vi "Calibration Helper2.vi"(7 "Std Devs":cluster{"H":dbl, "S":dbl, "V":dbl}={"H"=4.0, "S"=6.0, "V"=6.0}, 8 "Color Mode":u16(ring)=2 items=["RGB", "HSL", "HSV", "HSI", "CIE L*a*b*", "CIE XYZ"], 9 "Color Components":T1={"Hue"={110.0, 142.0}, "Sat"={138.0, 255.0}, "Val"={139.0, 198.0}} {"Val" scale=0.0..255.0; "Sat" scale=0.0..255.0; "Hue" scale=0.0..255.0 scale format="%#_3g"}, 10 "Image":T2, 11 "Image Ctl Refnum":refnum<vi>) -> (2 "Changed":bool, 3 "output color":T3)   [LabVIEW 2025]
doc: "Use the ROI (region of interest) to mask the image and compute a histogram of the indicated region. This provides the average H, S, and V values as well as the\nstandard deviation of each. It then calculates the initial upper and lower values we want to use for the threshold, and ensure that they are between 0 and 255. Hue, or the 0'th item is\na circular coordinate, so we sometimes flip the upper and lower when the computed value wraps past zero. The other values are linear and are simply clamped. This statistical approach is a reasonable approach when the ROI makes sense, but it is often useful to adjust the high/low values after the auto-calibration."
uses:
  <vilib>/vision/Image Controls.llb/IMAQ Image.ctl
  <vilib>/vision/NI_Vision_Development_Module.lvlib
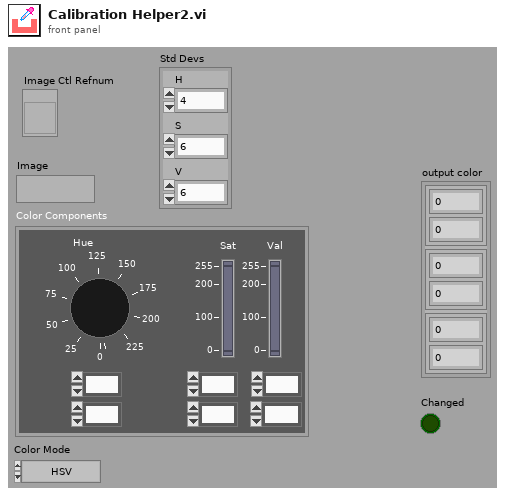
[diagram p1: front panel]
types:
  T1 = cluster{"Hue":cluster{dbl, dbl}, "Sat":cluster{dbl, dbl}, "Val":cluster{dbl, dbl}}
  T2 = typedef "IMAQ Image.ctl" = refnum<image>
  T3 = cluster{cluster{dbl, dbl}, cluster{dbl, dbl}, cluster{dbl, dbl}}
  T4 = typedef "Image Type" = u32
  T5 = cluster{"Global Rectangle":i32[], "Contours":cluster{"Contour Type":u32, "ROI Type":u32, "Points":i32[]}[]}
  T6 = cluster{"histogram":u32[], "Minimal Value":sgl, "Maximal Value":sgl, "Starting Value":sgl, "Interval Width":sgl, "Mean Value":sgl, "Standard  Variation":sgl, "Area (pixels)":i32}
  T7 = cluster{"histogram":u32[], "Minimal Value":sgl, "Maximal Value":sgl, "Starting Value":sgl, "Interval Width":sgl, "Mean Value":sgl, "Standard  Variation":sgl, "Area (pixels)":i32}[]
  T8 = cluster{"[0]":cluster{dbl, dbl}, "[1]":cluster{dbl, dbl}, "[2]":cluster{dbl, dbl}}
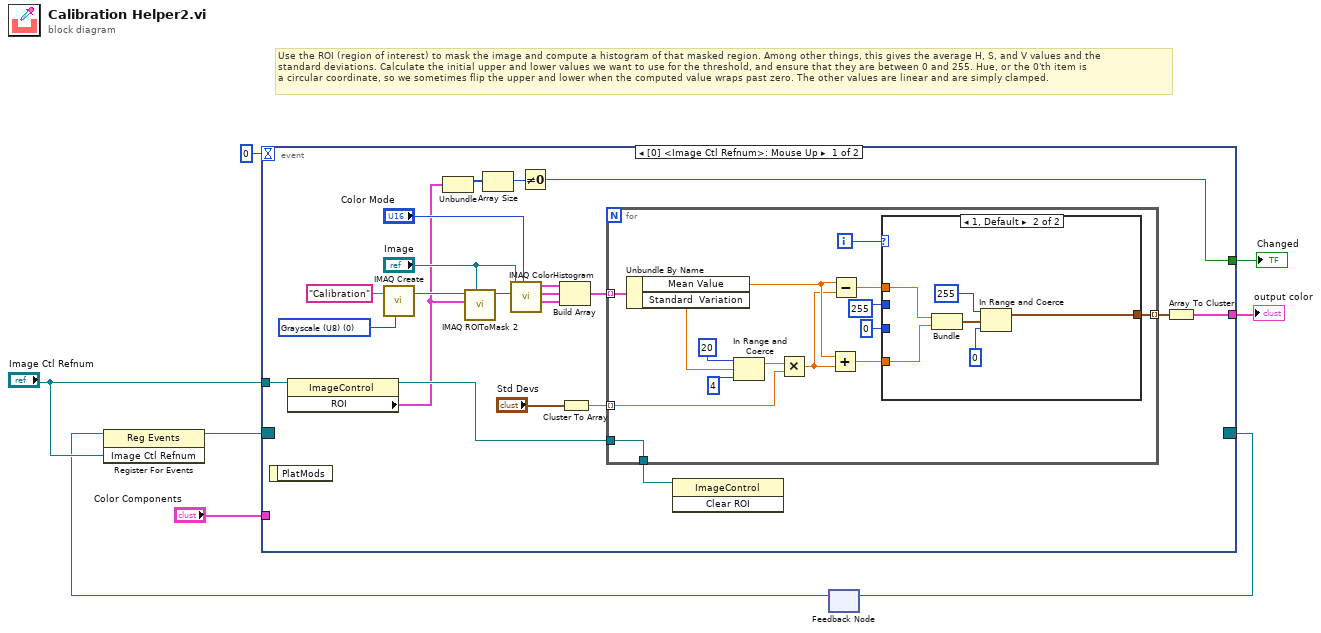
[diagram p0: block diagram]
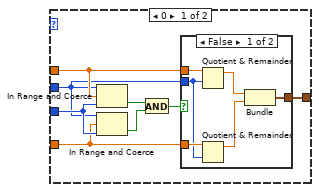
[diagram p2: hidden frame]
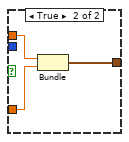
[diagram p3: hidden frame]
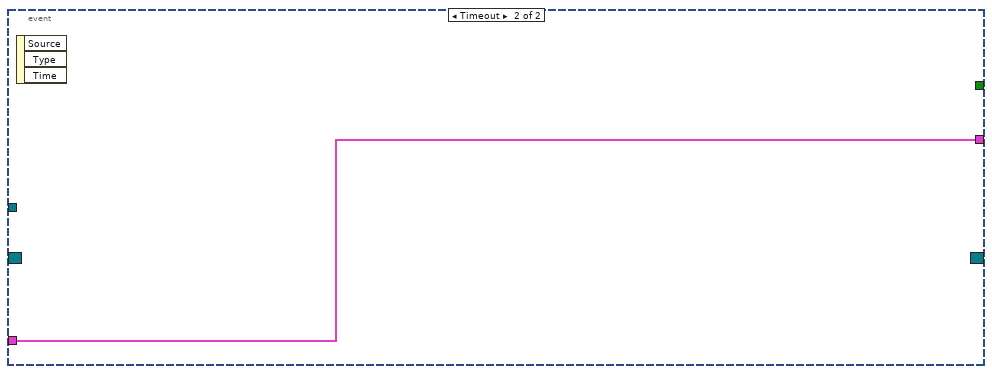
[diagram p4: hidden frame]
diagram:
  # "Use the ROI (region of interest) to mask the image and compute a histogram of that masked region. Among other things, this gives the average H, S, and V values and the\nstandard deviations. Calculate the initial upper and lower values we want to use for the threshold, and ensure that they are between 0 and 255. Hue, or the 0'th item is\na circular coordinate, so we sometimes flip the upper and lower when the computed value wraps past zero. The other values are linear and are simply clamped."
  n1 = feedback #1() -> (w2:refnum<event-registration>)  [unwired: 1 in]
  n2 = register-events(reference=w2, "Image Ctl Refnum") -> (reference out=w6:refnum<event-registration>)  [unwired: 1 in, 1 out]
  n3 = event shown="[0] <Image Ctl Refnum>: Mouse Up" {
    selector: w6 -> [_ _]
    dyn-events: [_ _] -> w3
    timeout: 0 -> [_ _]
    tunnel: "Image Ctl Refnum" -> [w16 _]
    tunnel: "Color Components" -> [_ w68]
    tunnel: [w13 w68] -> w4
    tunnel: [w9 _] -> w1
    event Mouse Up {
      w29 = T4 0 items=["Grayscale (U8)", "Grayscale (I16)", "Grayscale (SGL)", "Complex (CSG)", "RGB (U32)", "HSL (U32)", "RGB (U64)", "Grayscale (U16)"] ("Image Type")
      n4 = event-data() -> ()  [unwired: 1 in, 1 out]
      n5 = property on="Property Node" class="ImageControl"(reference=w16) -> (reference out=w14:refnum<vi>, "ROI"=w12:T5)  [unwired: 1 in, 1 out]
      n6 = call "IMAQ Create"("Image Name"="Calibration", "Image Type"=w29) -> ("New Image"=w26:T2)  [unwired: 3 in, 1 out]
      n7 = Unbundle(w12) -> ("Global Rectangle"=w11:i32[])  [unwired: 1 out]
      n8 = call "IMAQ ROIToMask 2"("Image Model"="Image", "ROI Descriptor"=w12, "Image"=w26) -> ("Image Out"=w27:T2)  [unwired: 6 in, 2 out]
      n9 = Array Size(array=w11) -> (size(s)=w10:i32)
      n10 = call "IMAQ ColorHistogram"("Color Mode"="Color Mode", "Image Src"="Image", "Image Mask"=w27) -> ("Red or Hue or X or L* Histogram Report"=w22:T6, "Green or Sat or Y or a* Histogram Report"=w21:T6, "Blue or Luma or Val or Inten or Z or b* Histogram Report"=w20:T6)  [unwired: 3 in, 1 out]
      n11 = Not Equal To 0?(x=w10) -> (x != 0?=w9:bool)
      n12 = Build Array(w22, w21, w20) -> (w18:T7)
      n13 = Cluster To Array(cluster="Std Devs") -> (array=w19:dbl[])
      n14 = for {
        tunnel: w19 -> [w40] mode=indexing
        tunnel: w18 -> [w44] mode=indexing
        tunnel: [w35] -> w17 mode=indexing
        tunnel: [w30] -> w15
        tunnel: w14 -> [w30]
        i -> [w33]
        n15 = Unbundle By Name(w44) -> ("Mean Value"=w38:sgl, "Standard  Variation"=w41:sgl)
        n16 = In Range and Coerce(upper limit=20, x=w41, lower limit=4) -> (coerced(x)=w39:sgl)  [unwired: 1 out]
        n17 = Multiply(x=w39, y=w40) -> (x*y=w34:dbl)
        n18 = Add(x=w38, y=w34) -> (x+y=w36:dbl)
        n19 = Subtract(x=w38, y=w34) -> (x-y=w37:dbl)
        n20 = case shown="1, Default" w33 {
          tunnel: w37 -> [w47 w64]
          tunnel: w36 -> [w46 w63]
          tunnel: [w49 w62] -> w35
          tunnel: 255 -> [w45 _]
          tunnel: 0 -> [w48 _]
          frame 0 {
            n21 = In Range and Coerce(upper limit=w45, x=w47, lower limit=w48) -> (In Range?=w51:bool)  [unwired: 1 out]
            n22 = In Range and Coerce(upper limit=w45, x=w46, lower limit=w48) -> (In Range?=w50:bool)  [unwired: 1 out]
            n23 = And(x=w51, y=w50) -> (x .and. y?=w52:bool)
            n24 = case shown="False" w52 {
              tunnel: [w55 w61] -> w49
              tunnel: w47 -> [w58 w59]
              tunnel: w46 -> [w57 w60]
              tunnel: w45 -> [w56 _]
              frame False {
                n25 = Quotient & Remainder(x=w58, y=w56) -> (x-y*floor(x/y)=w53:dbl)  [unwired: 1 out]
                n26 = Quotient & Remainder(x=w57, y=w56) -> (x-y*floor(x/y)=w54:dbl)  [unwired: 1 out]
                n27 = Bundle(w53, w54) -> (w55:cluster{dbl, dbl})  [unwired: 1 in]
              }
              frame True {
                n28 = Bundle(w59, w60) -> (w61:cluster{dbl, dbl})  [unwired: 1 in]
              }
            }
          }
          frame 1, Default {
            n29 = Bundle(w64, w63) -> (w67:cluster{dbl, dbl})  [unwired: 1 in]
            n30 = In Range and Coerce(upper limit=255, x=w67, lower limit=0) -> (coerced(x)=w62:cluster{dbl, dbl})  [unwired: 1 out]
          }
        }
      }
      n31 = invoke on="Invoke Node" class="ImageControl" method="Clear ROI"(reference=w15) -> ()  [unwired: 2 in, 3 out]
      n32 = Array To Cluster(array=w17) -> (cluster=w13:T8)
    }
    event Timeout {
      n33 = event-data() -> ()  [unwired: 1 in, 3 out]
    }
  }
  "output color" <- w4
  "Changed" <- w1
  n34 = feedback-in #1(w3) -> ()
